vi "I2C Communication.vi"(8 "error in":errorcluster) -> (0 "error out":errorcluster, 2 "Pass?":bool, 3 "VISA resource name out":refnum<visa-resource-name>)   [LabVIEW 2009]
uses:
  Digit IO PCI 6503/Digit IO control.ctl
  Global/Global 1.vi
  <vilib>/Instr/_visa.llb/VISA Configure Serial Port (Instr).vi
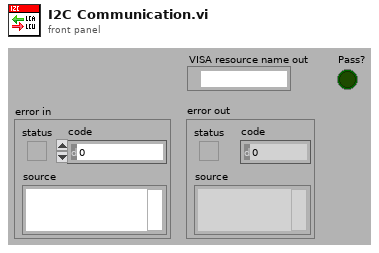
[diagram p1: front panel]
types:
  T1 = typedef "Digit IO control.ctl" = enum16{"Pull X1_4 Low", "Disconnect Pull X1_4 Low", "Down Cylinder", "Disconnect Down Cylinder", "Load X1_1_5", "Disconnect Load X1_1_5", "Measu X1_1_5", "Disconnect Measu X1_1_5", "Measu Z1_1_5", "Disconnect Measu Z1_1_5", "Power X1_1", "Disconnect Power X1_1", "RS232 Power", "Disconnect RS232 Power", "Card Cylinder", "Disconnect Card Cylinder", "Fail LED", "Disconnect Fail LED", "LCA Power", "Disconnect LCA Power", "BeyondCylinderDowndigit", "Disconnect BeyondCylinderDowendigit", "Frequency", "Disconnect Frequency", "Measu Current", "Disconnect Measu Current", "Measu current_1", "Disconnect Measu current_1", "Digit ALL", "Disconnect Digit ALL", "PASS LED", "Disconnect PASS LED", "Load Z1_1_3", "Disconnect Load Z1_1_3", "RS232 Connect", "Disconnect RS232 Connect", "Power Z1_7", "Disconnect Power Z1_7", "Pull Z_1_5  low", "Disconnect Pull Z_1_5  low", "Connect LCA_1", "Disconnect LCA_1", "short LCA", "Disconnect short LCA", "PT100", "Disconnect PT100", "NO connect", "Disconnect NO connect"}
  T2 = enum16{"LCA Power on", "Command _s", "Close Cylinder(LCA)", "Command _d", "Finish"}
  T3 = cluster{"People":string, "product  number":string, "Test time":string, "VHeatFuse_noload":string, "VHeatFuse_load":string, "VoverrideDiode":string, "Test firmware upload via X1":string, "TemperAddress":string, "Troom":string, "TLCU":string, "Adjustment factor":string, "MeasuredFreq":string, "I2C communication":string, "Light-emitting diode on Z2":string, "Battery warning/inhibit":string, "Reset by IC10":string, "External EEPROM":string, "RFID card detection and reading RFID":string, "Production parameters in internal EEPROM":string, "Current consumption in sleep mode":string, "Application and database upload":string, "Test result":string, "Table head[22]":string, "Table head[23]":string}
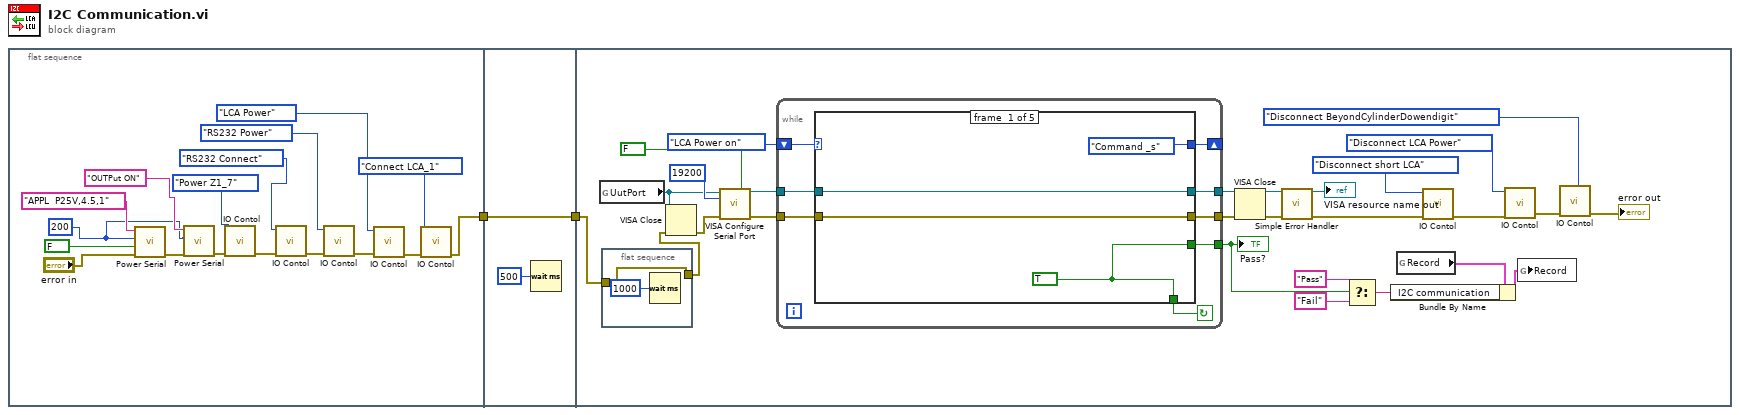
[diagram p0: block diagram]
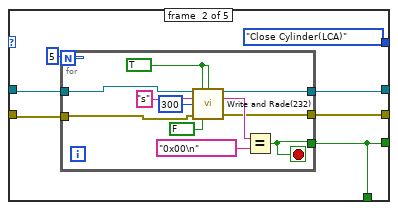
[diagram p2: hidden frame]
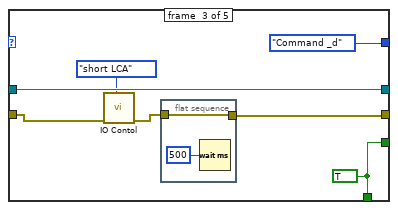
[diagram p3: hidden frame]
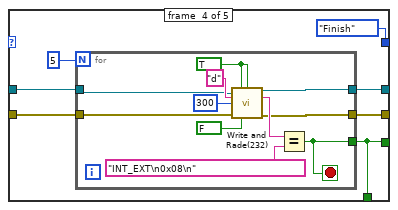
[diagram p4: hidden frame]
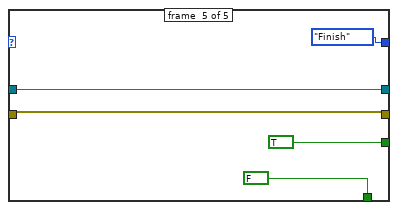
[diagram p5: hidden frame]
diagram:
  n1 = flat-sequence {
    tunnel: [w10] -> w2
    tunnel: w2 -> [w21]
    tunnel: [w21] -> w1
    tunnel: w1 -> [w30]
    frame #0 {
      w4 = 200 ("Delay")
      n2 = call "Power Serial.vi"("error in (no error)"="error in", "Rd?"=FALSE, "Delay"=w4, "IN"="APPL  P25V,4.5,1" ("In")) -> ("error out"=w6:errorcluster)  [unwired: 1 in, 6 out]
      n3 = call "Power Serial.vi"("error in (no error)"=w6, "Delay"=w4, "IN"="OUTPut ON" ("In")) -> ("error out"=w7:errorcluster)  [unwired: 2 in, 6 out]
      n4 = call "IO Contol.vi"("error in"=w7, "IO Operation"=Digit_IO_control."Power Z1_7" ("Enum")) -> ("error out"=w18:errorcluster)  [unwired: 9 out]
      n5 = call "IO Contol.vi"("error in"=w18, "IO Operation"=Digit_IO_control."RS232 Connect" ("Enum")) -> ("error out"=w19:errorcluster)  [unwired: 9 out]
      n6 = call "IO Contol.vi"("error in"=w19, "IO Operation"=Digit_IO_control."RS232 Power" ("Enum")) -> ("error out"=w14:errorcluster)  [unwired: 9 out]
      n7 = call "IO Contol.vi"("error in"=w14, "IO Operation"=Digit_IO_control."LCA Power") -> ("error out"=w12:errorcluster)  [unwired: 9 out]
      n8 = call "IO Contol.vi"("error in"=w12, "IO Operation"=Digit_IO_control."Connect LCA_1") -> ("error out"=w10:errorcluster)  [unwired: 9 out]
    }
    frame #1 {
      n9 = Wait (ms)(milliseconds to wait=u32 500) -> ()  [unwired: 1 out]
    }
    frame #2 {
      n10 = global read "Global 1.vi" "UutPort"() -> (w31:refnum<visa-resource-name>)
      n11 = flat-sequence {
        tunnel: w30 -> [w47]
        tunnel: [w47] -> w29
        frame #0 {
          n12 = Wait (ms)(milliseconds to wait=u32 1000) -> ()  [unwired: 1 out]
        }
      }
      n13 = VISA Close(VISA resource name=w31, error in (no error)=w29) -> (error out=w32:errorcluster)
      n14 = call-poly "VISA Configure Serial Port"("VISA resource name"=w31, "Enable Termination\nChar (T)"=FALSE ("Enable Termination\nChar (T)"), "baud rate (9600)"=u32 19200, "error in (no error)"=w32) -> ("VISA resource name out"=w39:refnum<visa-resource-name>, "error out"=w37:errorcluster)  [unwired: 3 in, 7 out]
      n15 = while {
        shift-right: [w49] -> _
        shift-left: T2."LCA Power on" -> [w56]
        tunnel: [w54] -> w40
        tunnel: w39 -> [w53]
        tunnel: [w52] -> w38
        tunnel: w37 -> [w51]
        tunnel: [w50] -> w35
        stop <- w55 continue-if-true
        n16 = case shown="\"Finish\"" w56 {
          tunnel: [T2."Command _s" T2."Close Cylinder(LCA)" T2."Command _d" T2."Finish" T2."Finish"] -> w49
          tunnel: [w58 w62 w83 w89 FALSE] -> w55
          tunnel: [w59 w63 w84 w91 w107] -> w54
          tunnel: w53 -> [w59 w66 w84 w93 w107]
          tunnel: [w57 w64 w79 w90 w106] -> w52
          tunnel: w51 -> [w57 w65 w81 w92 w106]
          tunnel: [w58 w62 w83 w89 TRUE] -> w50
          frame #0 {
            w58 = TRUE
          }
          frame #1 {
            n17 = for {
              N: 5 -> [_]
              tunnel: w66 -> [w69]
              tunnel: w65 -> [w68]
              tunnel: [w73] -> w64
              tunnel: [w72] -> w63
              tunnel: [w71] -> w62
              stop <- w71 stop-if-true
              w78 = TRUE ("write")
              n18 = call "Write and Rade(232).vi"("VISA resource name in"=w69, "write"=w78, "read"=w78, "string to write"="s", "ms delay"=u32 300 ("millisecond multiple"), "error in"=w68, "change baud rate(read)"=FALSE) -> ("VISA resource name out"=w72:refnum<visa-resource-name>, "read string"=w75:string, "error out"=w73:errorcluster)  [unwired: 1 in, 5 out]
              n19 = Equal?(x=w75, y="0x00\n") -> (x = y?=w71:bool)
            }
          }
          frame #2 {
            w83 = TRUE
            n20 = call "IO Contol.vi"("error in"=w81, "IO Operation"=Digit_IO_control."short LCA") -> ("error out"=w80:errorcluster)  [unwired: 9 out]
            n21 = flat-sequence {
              tunnel: w80 -> [w87]
              tunnel: [w87] -> w79
              frame #0 {
                n22 = Wait (ms)(milliseconds to wait=u32 500) -> ()  [unwired: 1 out]
              }
            }
          }
          frame #3 {
            n23 = for {
              N: 5 -> [_]
              tunnel: w93 -> [w96]
              tunnel: w92 -> [w95]
              tunnel: [w100] -> w91
              tunnel: [w99] -> w90
              tunnel: [w98] -> w89
              stop <- w98 stop-if-true
              w105 = TRUE ("write")
              n24 = call "Write and Rade(232).vi"("VISA resource name in"=w96, "write"=w105, "read"=w105, "string to write"="d", "ms delay"=u32 300 ("millisecond multiple"), "error in"=w95, "change baud rate(read)"=FALSE) -> ("VISA resource name out"=w100:refnum<visa-resource-name>, "read string"=w102:string, "error out"=w99:errorcluster)  [unwired: 1 in, 5 out]
              n25 = Equal?(x=w102, y="INT_EXT\n0x08\n") -> (x = y?=w98:bool)
            }
          }
          frame #4 {
          }
        }
      }
      "VISA resource name out" <- w40
      "Pass?" <- w35
      n26 = VISA Close(VISA resource name=w40, error in (no error)=w38) -> (error out=w42:errorcluster)
      n27 = call <vilib>:"Simple Error Handler.vi"("error in (no error)"=w42) -> ("error out"=w27:errorcluster)  [unwired: 1 in, 7 out]
      n28 = Select(t="Pass", s=w35, f="Fail") -> (s? t:f=w34:string)
      n29 = global read "Global 1.vi" "Record"() -> (w46:T3)
      n30 = Bundle By Name(cluster=w46, "I2C communication"=w34) -> (w45:T3)
      n31 = call "IO Contol.vi"("error in"=w27, "IO Operation"=Digit_IO_control."Disconnect short LCA") -> ("error out"=w23:errorcluster)  [unwired: 9 out]
      n32 = call "IO Contol.vi"("error in"=w23, "IO Operation"=Digit_IO_control."Disconnect LCA Power") -> ("error out"=w26:errorcluster)  [unwired: 9 out]
      n33 = global write "Global 1.vi" "Record"(w45) -> ()
      n34 = call "IO Contol.vi"("error in"=w26, "IO Operation"=Digit_IO_control."Disconnect BeyondCylinderDowendigit") -> ("error out"=→"error out":errorcluster)  [unwired: 9 out]
    }
  }
